vi "CSM - Populate Configuration Variables.vi"(5 "Section Name(\"\" as Default)":string, 7 "error in (no error)":errorcluster, 9 "String in":string) -> (1 "error out":errorcluster, 3 "String out":string)   [LabVIEW 2017, in "INI-Static-Variable-Support.lvlib"]
uses:
  INI-Static-Variable-Support.lvlib
  <userlib>/_NEVSTOP/Communicable State Machine(CSM)/_Support/ChangeFlag/ChangeFlag-Read.vi
  <userlib>/_NEVSTOP/Communicable State Machine(CSM)/_Support/ChangeFlag/ChangeFlagDB.vi
  <userlib>/_NEVSTOP/Communicable State Machine(CSM)/Communicable State Machine.lvlib
  <userlib>/_NEVSTOP/Communicable State Machine(CSM)/_Shared/CSM Shared.lvlib
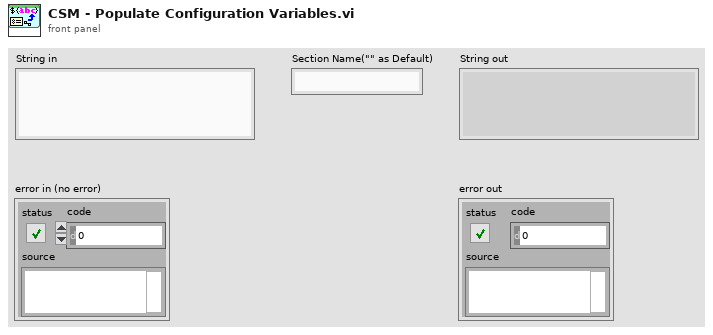
[diagram p1: front panel]
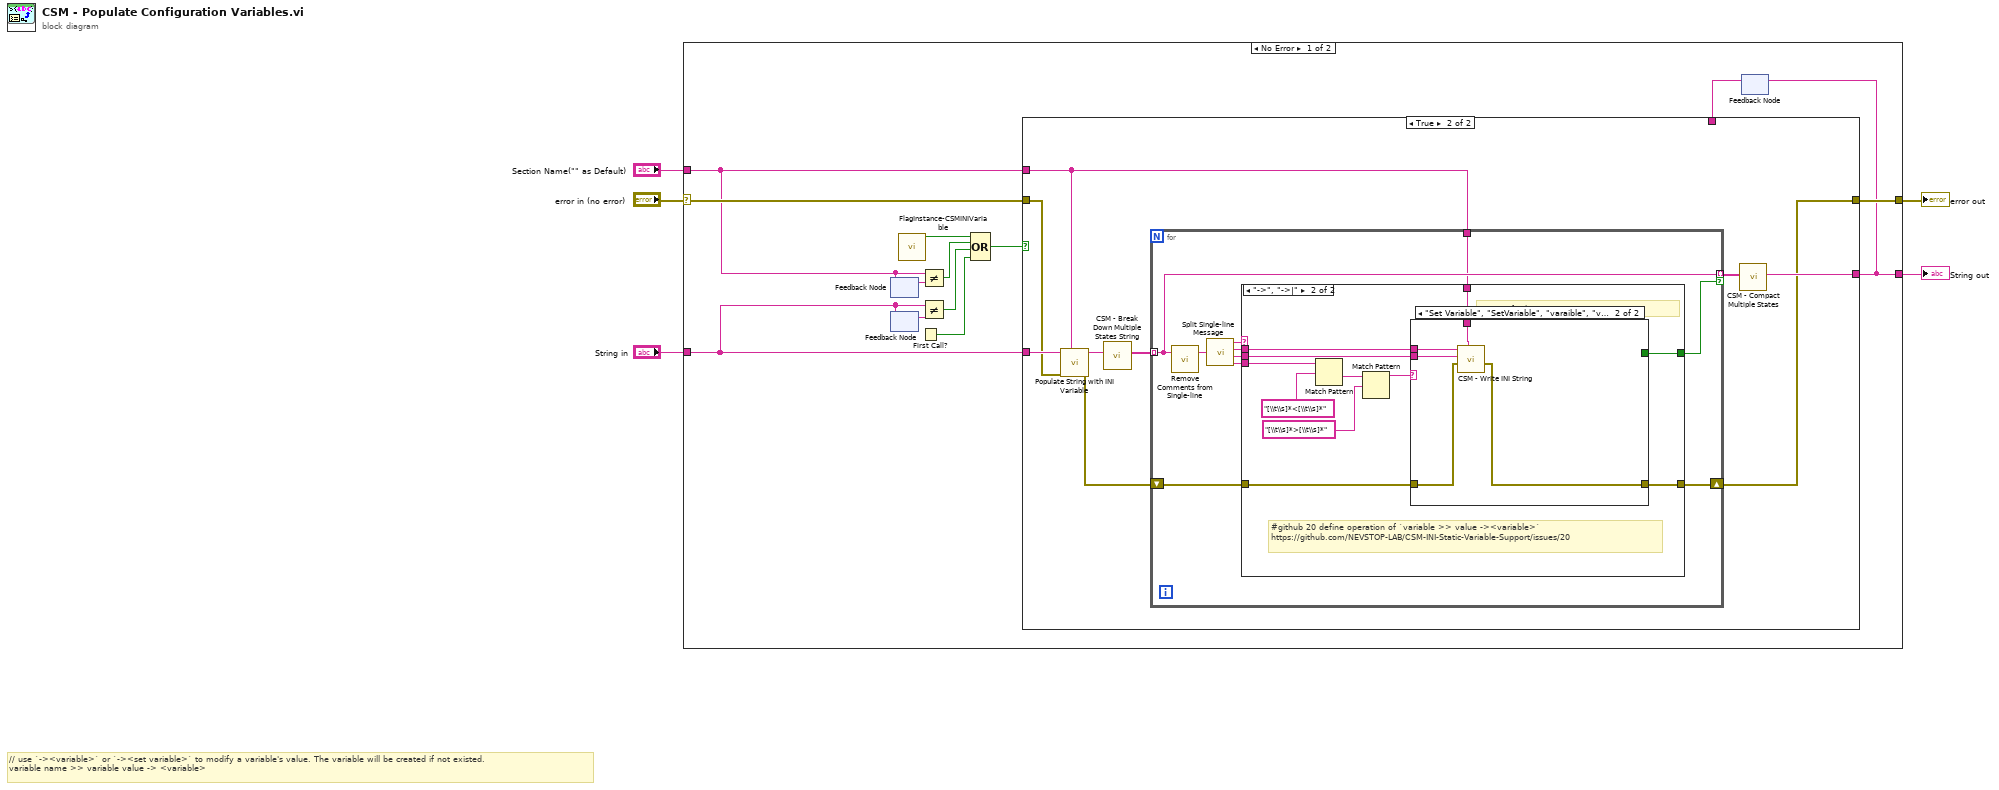
[diagram p0: block diagram]
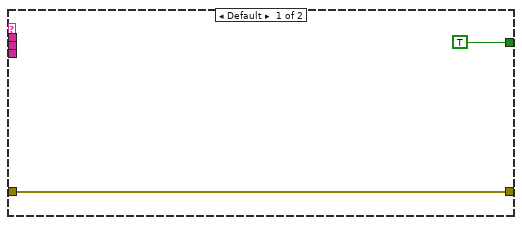
[diagram p3: hidden frame]
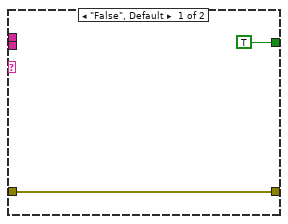
[diagram p4: hidden frame]
diagram:
  # "// use `-><variable>` or `-><set variable>` to modify a variable's value. The variable will be created if not existed.\nvariable name >> variable value -> <variable>"
  n1 = case shown="No Error" "error in (no error)" {
    selector: "error in (no error)" -> [w17 w61]
    tunnel: [w18 w61] -> w5
    tunnel: "String in" -> [w11 _]
    tunnel: "Section Name(\"\" as Default)" -> [w10 w60]
    tunnel: [w8 w60] -> w1
    frame No Error {
      n2 = feedback #1() -> (w16:string)  [unwired: 1 in]
      n3 = feedback-in #1(w10) -> ()
      n4 = feedback #2() -> (w15:string)  [unwired: 1 in]
      n5 = feedback-in #2(w11) -> ()
      n6 = call "FlagInstance-CSMINIVariable.vi"() -> ("Changed"=w6:bool)  [unwired: 10 in, 1 out]
      n7 = First Call?() -> (First Call?: T/F=w12:bool)
      n8 = Not Equal?(x=w10, y=w16) -> (x != y?=w14:bool)
      n9 = Not Equal?(x=w11, y=w15) -> (x != y?=w13:bool)
      n10 = Compound Arithmetic op=OR(w6, w14, w13, w12) -> (w9:bool)
      n11 = feedback #3() -> (w7:string)  [unwired: 1 in]
      n12 = case shown="True" w9 {
        tunnel: [w20 w21] -> w18
        tunnel: w17 -> [w20 w22]
        tunnel: [w19 w26] -> w8
        tunnel: w11 -> [_ w24]
        tunnel: w10 -> [_ w23]
        tunnel: w7 -> [w19 _]
        frame False {
        }
        frame True {
          n13 = call "Populate String with INI Variable.vi"("Section"=w23, "Error in"=w22, "String might with variables"=w24) -> ("Error out"=w25:errorcluster, "String out"=w28:string)  [unwired: 5 in]
          n14 = call <userlib>:"CSM - Break Down Multiple States String.vi"("States"=w28) -> ("Multiple States"=w29:string[])  [unwired: 10 in]
          n15 = for {
            tunnel: w29 -> [w34] mode=indexing
            tunnel: [w34] -> w27 mode=indexing if=w33
            tunnel: w23 -> [w32]
            shift-right: [w31] -> w21
            shift-left: w25 -> [w30]
            n16 = call <userlib>:"Remove Comments from Single-line.vi"("single-line text"=w34) -> ("single-line text without comments"=w39:string)  [unwired: 2 in]
            n17 = call <userlib>:"Split Single-line Message.vi"("single-line text"=w39) -> ("operator"=w38:string, "state"=w36:string, "args"=w35:string, "source/target"=w37:string)  [unwired: 6 in]
            n18 = case shown="\"->\", \"->|\"" w38 {
              tunnel: w37 -> [_ w52]
              tunnel: w36 -> [_ w47]
              tunnel: w35 -> [_ w46]
              tunnel: [TRUE w45] -> w33
              tunnel: w32 -> [_ w44]
              tunnel: [w40 w43] -> w31
              tunnel: w30 -> [w40 w42]
              frame Default {
              }
              frame "->", "->|" {
                # "#github 20 define operation of `variable >> value -><variable>`\nhttps://github.com/NEVSTOP-LAB/CSM-INI-Static-Variable-Support/issues/20"
                # "typo to for better customer experience"
                n19 = Match Pattern(string=w52, regular expression="[\\t\\s]*<[\\t\\s]*") -> (after substring=w49:string)  [unwired: 1 in, 3 out]
                n20 = Match Pattern(string=w49, regular expression="[\\t\\s]*>[\\t\\s]*") -> (before substring=w48:string)  [unwired: 1 in, 3 out]
                n21 = case shown="\"Set Variable\", \"SetVariable\", \"varaible\", \"variable\"" w48 {
                  tunnel: w47 -> [_ w59]
                  tunnel: w46 -> [_ w58]
                  tunnel: [TRUE _] -> w45
                  tunnel: w44 -> [_ w57]
                  tunnel: [w53 w55] -> w43
                  tunnel: w42 -> [w53 w56]
                  frame "False", Default {
                  }
                  frame "Set Variable", "SetVariable", "varaible", "variable" {
                    n22 = call "CSM - Write INI String.vi"("Section Name(\"\" as Default)"=w57, "error in (no error)"=w56, "String"=w58, ">> Variable Name >>"=w59) -> ("error out"=w55:errorcluster)  [unwired: 4 in, 1 out]
                  }
                }
              }
            }
          }
          n23 = call <userlib>:"CSM - Compact Multiple States.vi"("Multiple States"=w27) -> ("States"=w26:string)  [unwired: 9 in]
        }
      }
      n24 = feedback-in #3(w8) -> ()
    }
    frame Error {
    }
  }
  "error out" <- w5
  "String out" <- w1
